vi "Last Ack Creator Queue.vi"(10 "Queue":refnum<class "Queue.lvclass">) -> (2 "Msg Strategy":refnum<class "Msg Strategy.lvclass">)   [LabVIEW 2021, in "jettl.lvlib" / "Last Ack Creator Queue Msg Strategy.lvlib"]
uses:
  Last Ack Creator Queue Msg Strategy.lvlib
  Msg Strategy/Msg Strategy.lvclass
  Queue/Queue.lvclass
  Last Ack Creator Queue Msg Strategy/Last Ack Creator Queue Msg Strategy.lvclass
  C:/git/jettl/jettl/jettl/Msg Strategy/Msg Strategy.lvclass
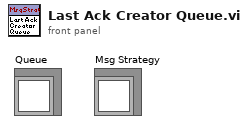
[diagram p1: front panel]
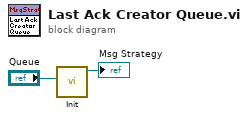
[diagram p0: block diagram]
diagram:
  n1 = call "Init.vi"("Queue"="Queue") -> ("Last Ack Creator Queue Msg Strategy out"=→"Msg Strategy":refnum<class "Last Ack Creator Queue Msg Strategy.lvclass">)  [unwired: 10 in]
